vi "SendTelnetCmds.vi"(2 "error in":errorcluster, 3 "Write_strings":T1(array[cluster])=[{"WriteData"="\n", "DelayAfterWrite"=1000.0}, {"WriteData"="uci show skywire\n", "DelayAfterWrite"=1000.0}], 5 "Target IP":string="66.212.64.194") -> (0 "error out":errorcluster, 1 "Response":string[](array[string])=["                === IMPORTANT ============================    Use 'passwd' to set your login password    this will disable telnet and enable SSH   ------------------------------------------      BusyBox v1.22.1 (2015-03-30 15:58:59 CDT) built-in shell (ash)  Enter 'help' for a list of built-in commands.      _______                     ________        __   |       |.-----.-----.-----.|  |  |  |.----.|  |_   |   -   ||  _  |  -__|     ||  |  |  ||   _||   _|   |_______||   __|_____|__|__||________||__|  |____|            |__| W I R E L E S S   F R E E D O M   -----------------------------------------------------   BARRIER BREAKER (Barrier Breaker, r44952)   -----------------------------------------------------    * 1/2 oz Galliano         Pour all ingredients into    * 4 oz cold Coffee        an irish coffee mug filled    * 1 1/2 oz Dark Rum       with crushed ice. Stir.    * 2 tsp. Creme de Cacao   -----------------------------------------------------  root@OpenWrt:/#   root@OpenWrt:/# ", " "])   [LabVIEW 2013]
doc: "This VI implements a client for the named service created by Named Service TCP Server.vi.\nThe client connects to the service using the name of the service and the address of the server. It receives the response from the server, displays it and closes the connection.\n\n<b>Note:</b> This VI is built to work with the Named Service TCP Server.vi in TCP.llb."
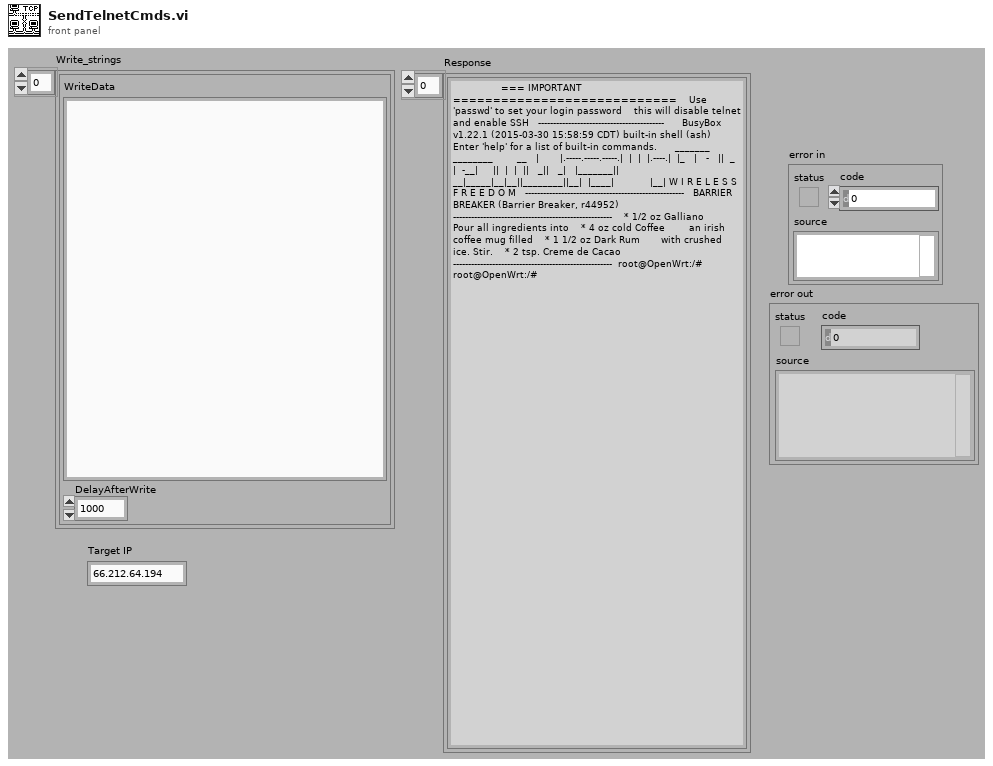
[diagram p1: front panel]
types:
  T1 = cluster{"WriteData":string, "DelayAfterWrite":dbl}[]
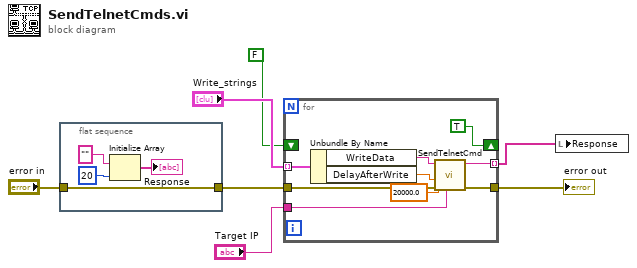
[diagram p0: block diagram]
diagram:
  n1 = flat-sequence {
    tunnel: [w8] -> w4
    tunnel: "error in" -> [w8]
    frame #0 {
      n2 = Initialize Array("", 20 ("dimension size")) -> (→"Response":string[])
    }
  }
  n3 = for {
    tunnel: "Write_strings" -> [w20] mode=indexing
    tunnel: "Target IP" -> [w19]
    tunnel: w4 -> [w17]
    tunnel: [w16] -> w2
    shift-right: [TRUE ("Use existing connection?")] -> _
    shift-left: FALSE ("Use existing connection?") -> [_]
    tunnel: [w14] -> w1 mode=indexing
    n4 = Unbundle By Name(w20) -> ("WriteData"=w13:string, "DelayAfterWrite"=w18:dbl)
    n5 = call "SendTelnetCmd.vi"("Target IP"=w19, "error in"=w17, "DelayAfterWrite"=w18, "Initial delay"=20000.0, "WriteData"=w13) -> ("error out"=w16:errorcluster, "Response"=w14:string)  [unwired: 5 in]
  }
  "error out" <- w2
  n6 = local write "Response"(w1) -> ()
